vi "Enter set temperature safety delta in Celcius.vi"() -> ()   [LabVIEW 2018, in "Hei-End.lvlib"]
uses:
  <instrlib>/Hei-End/Hei-End.lvlib
panel:
  out "error out":errorcluster
  out "VISA resource name out":refnum<visa-resource-name>
  in  "Temperature (C)":dbl
  in  "error in (no error)":errorcluster
  in  "VISA resource name":refnum<visa-resource-name>
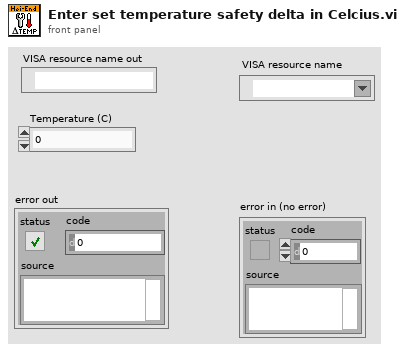
[diagram p1: front panel]
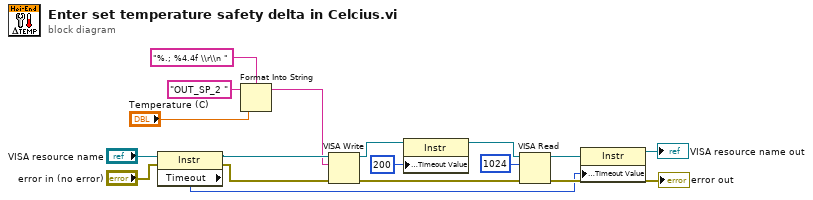
[diagram p0: block diagram]
diagram:
  n1 = property class="Instr"(reference="VISA resource name", error in="error in (no error)") -> (reference out=w4:refnum<visa-resource-name>, error out=w3:errorcluster, "Timeout"=w2:u32)
  n2 = Format Into String(format string="%.; %4.4f \\r\\n ", initial string="OUT_SP_2 ", "Temperature (C)") -> (resulting string=w1:string)  [unwired: 1 in, 1 out]
  n3 = VISA Write(VISA resource name=w4, write buffer=w1, error in (no error)=w3) -> (VISA resource name out=w6:refnum<visa-resource-name>, error out=w9:errorcluster)  [unwired: 1 out]
  n4 = property class="Instr"(reference=w6, "General Settings:Timeout Value"=u32 200) -> (reference out=w5:refnum<visa-resource-name>)  [unwired: 1 in, 1 out]
  n5 = VISA Read(VISA resource name=w5, byte count=u32 1024, error in (no error)=w9) -> (VISA resource name out=w10:refnum<visa-resource-name>, error out=→"error out":errorcluster)  [unwired: 2 out]
  n6 = property class="Instr"(reference=w10, "General Settings:Timeout Value"=w2) -> (reference out=→"VISA resource name out":refnum<visa-resource-name>)  [unwired: 1 in, 1 out]
